vi "SQLSTATE Lookup.vi"(4 "SQLSTATE Value":string) -> (1 "SQLSTATE Description":string)   [LabVIEW 2014, in "hse-db.lvlib" / "ADO-DB-Driver.lvlib"]
uses:
  ADO-DB-Driver.lvlib
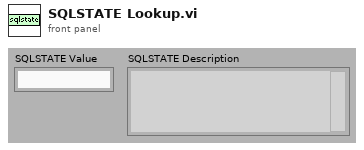
[diagram p1: front panel]
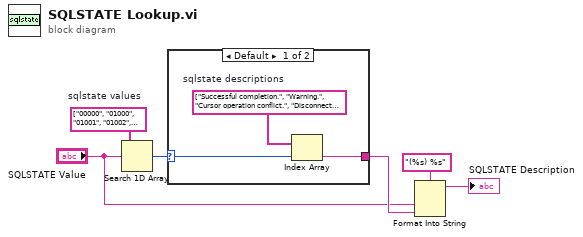
[diagram p0: block diagram]
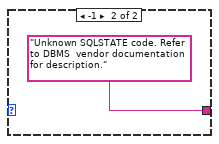
[diagram p2: hidden frame]
diagram:
  w6 = string[] ["00000", "01000", "01001", "01002", "01003", "01004", "01006", "01007", "01008", "01009", "0100A", "0100C", "0100D", "0100E", "01503", "01504", "01505", "01506", "01515", "01517", "01519", "01520", "01522", "01526", "01528", "01532", "01534", "01535", "01536", "01539", "01542", "01544", "01545", "01547", "01548", "01557", "01564", "01565", "01567", "01587", "01593", "01594", "01627", "01634", "01643", "01646", "01647", "01658", "01660", "01662", "02000", "02001", "07000", "07001", "07002", "07003", "07004", "07005", "07006", "07007", "07008", "07009", "08000", "08001", "08002", "08003", "08004", "08006", "08007", "09000", "0A000", "0A001", "0E000", "0F001", "0K000", "0W000", "0Z001", "0Z002", "20000", "21000", "22000", "22001", "22002", "22003", "22004", "22005", "22006", "22007", "22008", "22009", "22011", "22012", "22015", "22018", "22019", "22021", "22022", "22023", "22024", "22025", "22026", "22027", "22501", "22503", "22504", "22511", "22522", "22524", "22525", "23000", "23001", "23502", "23503", "23504", "23505", "23511", "23512", "23513", "23515", "23520", "23522", "24000", "24501", "24502", "24504", "24506", "24507", "24513", "24514", "25000", "25006", "25501", "26000", "26501", "26510", "27000", "28000", "2A000", "2B000", "2C000", "2D000", "2E000", "2D522", "2D528", "2D529", "2E000", "2F002", "2F003", "2F004", "2F005", "33000", "34000", "35000", "36001", "37000", "38001", "38002", "38003", "38004", "38501", "39004", "3B001", "3B002", "3B501", "3B502", "3C000", "3D000", "3F000", "40000", "40001", "40002", "40003", "42000", "42501", "42502", "42506", "42601", "42602", "42603", "42604", "42605", "42606", "42607", "42609", "42610", "42611", "42612", "42613", "42614", "42615", "42616", "42617", "42618", "42620", "42621", "42622", "42623", "42625", "42629", "42631", "42701", "42702", "42703", "42704", "42705", "42707", "42709", "42710", "42711", "42712", "42713", "42718", "42723", "42724", "42725", "42726", "42732", "42733", "42734", "42736", "42737", "42738", "42802", "42803", "42804", "42805", "42806", "42807", "42808", "42809", "42810", "42811", "42812", "42813", "42814", "42815", "42816", "42817", "42818", "42819", "42820", "42821", "42822", "42823", "42824", "42825", "42826", "42827", "42828", "42829", "42830", "42832", "42833", "42834", "42835", "42836", "42837", "42841", "42842", "42845", "42846", "42847", "42848", "42850", "42851", "42852", "42854", "42855", "42857", "42858", "42860", "42862", "42863", "42866", "42872", "42873", "42874", "42875", "42876", "42877", "42878", "42879", "42880", "42881", "42882", "42883", "42884", "42885", "42886", "42887", "42888", "42889", "42890", "42891", "42892", "42893", "42894", "42895", "42896", "42898", "42899", "428A1", "428B3", "428B7", "428B8", "428BA", "428C1", "428C7", "428C9", "428D1", "428D2", "428D4", "428D5", "428D6", "428D7", "428D8", "428EC", "428EK", "428EW", "428F1", "428F2", "428F9", "428FA", "428FC", "428FD", "428FE", "428FR", "428FT", "428FY", "428G0", "428G2", "42903", "42904", "42906", "42907", "42908", "42910", "42911", "42912", "42914", "42917", "42918", "42919", "42922", "42923", "42924", "42926", "42929", "42930", "42932", "42937", "42939", "42944", "42961", "42962", "42969", "42970", "42971", "42972", "42977", "42978", "42981", "42984", "42985", "42987", "42990", "42995", "42996", "42998", "42999", "429B6", "429B7", "429BD", "429BH", "429BM", "44000", "46001", "46002", "46003", "46007", "46008", "46501", "51002", "51003", "51004", "51009", "51015", "51021", "51035", "51036", "51037", "51039", "53038", "53039", "53045", "54001", "54002", "54004", "54005", "54006", "54008", "54009", "54010", "54011", "54018", "54019", "54021", "54023", "54028", "54035", "54038", "54044", "54054", "55005", "55006", "55007", "55018", "55019", "55029", "55042", "55048", "55050", "56016", "56084", "56095", "560BF", "560C4", "57005", "57006", "57007", "57011", "57012", "57013", "57014", "57017", "57033", "57042", "57043", "57050", "58003", "58004", "58008", "58009", "58010", "58011", "58012", "58014", "58015", "58016", "58017", "58018", "58028", "58033", "60000", "61000", "62000", "63000", "64000", "65000", "66000", "67000", "69000", "72000", "82100", "82101", "82102", "82103", "82104", "82105", "82106", "82107", "82108", "82109", "82110", "82111", "82112", "82113", "82114", "82115", "82116", "82117", "82118", "82119", "82120", "82121", "82122", "90000", "99999", "HZ000"]  # sqlstate values
  n1 = Search 1D Array(1D array=w6, element="SQLSTATE Value") -> (index of element=w1:i32)  [unwired: 1 in]
  n2 = case shown="Default" w1 {
    selector: w1 -> [w7 _]
    tunnel: [w8 "Unknown SQLSTATE code. Refer to DBMS  vendor documentation for description."] -> w5
    frame Default {
      w9 = string[] ["Successful completion.", "Warning.", "Cursor operation conflict.", "Disconnect error.", "Null value eliminated in set function.", "The value of a string was truncated when assigned to another string data type with a shorter length.", "Privilege not revoked.", "Privilege not granted.", "Implicit zero-bit padding.", "Search condition too long for information schema.", "Query expression too long for information schema.", "One or more ad hoc result sets were returned from the procedure.", "The cursor that was closed has been reopened on the next result set within the chain.", "The procedure returned too many result sets.", "The number of result columns is larger than the number of host variables provided.", "The update or delete statement does not include a where clause.", "The statement was not executed because it is unacceptable in this environment.", "An adjustment was made to a date or timestamp value to correct an invalid date resulting from an arithmetic operation.", "The null value has been assigned to a host variable, because the non-null value of the column is not within the range of the host variable.", "A character that cannot be converted was replaced with a substitute character.", "The null value has been assigned to a host variable, because a numeric value is out of range.", "The null value has been assigned to a host variable, because the characters cannot be converted.", "The local table or view name used in the \"create alias\" statement is undefined.", "Isolation level has been escalated.", "Where not null is ignored, because the index key cannot contain null values.", "An undefined object name was detected.", "The string representation of a datetime value is invalid.", "An arithmetic operation on a date or timestamp has a result that is not within the valid range of dates.", "During remote bind where existence checking is deferred, the server-name specified does not match the current server.", "Connection is successful but only sbcs characters should be used.", "Authorization id does not have the privilege to perform the operation as specified.", "The null value has been assigned to a host variable, because a substring error occurred; for example, an argument of substr is out of range.", "An unqualified column name has been interpreted as a correlated reference.", "A mixed data value is improperly formed.", "The authorization id does not have the privilege to perform the specified operation on the identified object.", "Too many host variables have been specified on select into or fetch.", "The null value has been assigned to a host variable, because division by zero occurred.", "The null value has been assigned to a host variable, because a miscellaneous data exception occurred; for example, the character value for the cast, decimal, float, or integer scalar function is invalid; a floating-point NaN (not a number) or invalid data in a packed decimal field was detected.", "The table was created but not journaled.", "The unit of work was committed or rolled back, but the outcome is not fully known at all sites.", "An alter table may cause data truncation.", "Insufficient number of entries in an SQLDA for all information (i.e. Not enough descriptors to return the distinct name).", "The datalink value may not be valid because the table is in reconcile pending or reconcile is not a possible state.", "The distinct data type name is too long and cannot be returned in the SQLDA. The short name is returned instead.", "Assignment to SQLCODE or SQLSTATE variable does not signal a warning or error.", "A result sets cannot be returned because the cursor was closed.", "A db2sql before trigger changed to db2row.", "Binary data is invalid for decrypt_char and decyrypt_db.", "The routine was created but a restore will not update the catalog.", "Release record option ignored on close.", "No data found.", "No additional result sets returned.", "Dynamic SQL error.", "The number of host variables is not correct for the number of parameter markers.", "The call parameter list is invalid.", "Cursor specification cannot be executed.", "Using clause required for dynamic parameters.", "Prepared statement not a cursor specification.", "Restricted datatype attribute violation.", "Using clause required for result fields.", "Invalid descriptor count.", "Invalid descriptor index.", "Connection exception.", "Client is unable to establish a connection.", "Connection name in use.", "Connection does not exist.", "The server rejected the connection.", "Connection failure.", "Transaction resolution unknown.", "A triggered SQL statement failed.", "Feature not supported.", "Multiple server transactions.", "The schema name list in a set(tm) path statement is not valid.", "The locator value does not currently represent any value.", "A resignal was issued but a handler is not active.", "The statement is not allowed in a trigger.", "Maximum number of stacked diagnostics areas exceeded.", "Stacked diagnostics accessed without and active handler.", "The case was not found for the case statement.", "The result of a select into, scalar fullselect, or subquery of a basic predicate is more than one value.", "Data exception.", "String data truncated (on right) on insert or update.", "Null value returned with no indicator variable provided.", "Numeric value out-of-range or overflow.", "A null value cannot returned from a procedure that is defined as parameter style general or a type-preserving method that is invoked with a non-null argument.", "Error in assignment.", "The fetch orientation is invalid.", "Invalid date-time format.", "Date-time field overflow.", "Invalid time zone displacement value.", "Substring error.", "Divide by zero error.", "Interval field overflow.", "Invalid character value for cast.", "Invalid escape character (in the \"like\" predicate?).", "A character is not in the coded character set or the conversion is not supported.", "Indicator variable overflow.", "Invalid parameter value.", "Unterminated C string passed as input host variable.", "Invalid escape sequence, for example, escape char not followed by %, _, or escape char.", "String data - length mismatch.", "Trim error.", "The length control field of a variable length string is negative or greater than the maximum.", "The string representation of a name is invalid.", "A mixed data value is invalid.", "ADT length exceeds maximum column length. The value for a rowid or reference column is not valid.", "A ccsid value is not valid at all, not valid for the data type or subtype, or not valid for the encoding scheme.", "Character conversion resulted in truncation.", "Partitioning key value is not valid.", "Integrity constraint violation.", "The update or delete of a parent key is prevented by a restrict update or delete rule.", "An insert or update value is null, but the column cannot contain null values.", "The insert or update value of a foreign key is invalid.", "The update or delete of a parent key is prevented by a no action update or delete rule.", "A violation of the constraint imposed by a unique index or a unique constraint occurred.", "A parent row cannot be deleted, because the check constraint restricts the deletion.", "The check constraint cannot be added, because the table contains rows that do not satisfy the constraint definition.", "The resulting row of the insert or update does not conform to the check constraint definition.", "The unique index cannot be created or unique constraint added because the table contains duplicate values of the specified key.", "The foreign key cannot be defined, because all of its values are not equal to a parent key of the parent table.", "The range of values for the identity column or sequence is exhausted.", "Invalid cursor state.", "The identified cursor is not open.", "The cursor identified in an open statement is already open.", "The cursor identified in the update, delete, set, or get statement is not positioned on a row.", "The statement identified in the prepare is the statement of an open cursor.", "Fetch current was specified, but the current row is deleted, or a value of an order by column of the current row has changed.", "Fetch next, prior, current, or relative is not allowed, because the cursor position is not known.", "A previous error has disabled this cursor.", "Invalid transaction state.", "An update operation is not valid because the transaction is read only.", "The statement is only allowed as the first statement in a unit of work.", "Invalid SQL statement name.", "The statement identified does not exist.", "The statement name specified in a declare cursor already has a cursor allocated to it.", "Triggered data change violation.", "Invalid authorization specification.", "Direct SQL syntax error or access rule violation.", "Dependent privilege descriptors still exist.", "Invalid character set name.", "Invalid transaction termination.", "Invalid connection name.", "Commit and rollback are not allowed in an atomic compound statement.", "Dynamic commit or commit on return procedure is invalid for the application execution environment.", "Dynamic rollback is invalid for the application execution environment.", "Connection name is invalid.", "The SQL function attempted to modify data, but the function was not defined as modifies SQL data.", "The statement is not allowed in a function or procedure.", "The SQL function attempted to read data, but the function was not defined as reads SQL data.", "The function did not execute a return statement.", "Invalid SQL descriptor name.", "Invalid cursor name.", "Invalid condition number.", "A sensitive cursor cannot be defined for the specified select-statement.", "Dynamic SQL syntax error or access rule violation.", "The external routine is not allowed to execute SQL statements.", "The external routine attempted to modify data, but the routine was not defined as modifies SQL data.", "The statement is not allowed in a routine.", "The external routine attempted to read data, but the routine was not defined as reads SQL data.", "Error occurred while calling a user-defined function, external procedure, or trigger (using the simple call or simple call with nulls calling convention).", "A null value is not allowed for an in or inout argument when using parameter style general or an argument that is a java(tm) primitive type.", "The savepoint is not valid.", "The maximum number of savepoints has been reached.", "A duplicate savepoint name was detected.", "A release or rollback to savepoint was specified, but a savepoint does not exist.", "Ambiguous cursor name.", "Invalid catalog name.", "Invalid schema name.", "Transaction rollback.", "Serialization failure. Transaction rollback due to deadlock.", "Integrity constraint violation.", "Statement completion unknown.", "Syntax error or access rule violation.", "The authorization id does not have the privilege to perform the specified operation on the identified object.", "The authorization id does not have the privilege to perform the operation as specified.", "Owner authorization failure occurred.", "A character, token, or clause is invalid or missing.", "A character that is invalid in a name has been detected.", "An unterminated string constant has been detected.", "An invalid numeric or string constant has been detected.", "The number of arguments specified for a scalar function is invalid.", "An invalid hexadecimal constant has been detected.", "An operand of a column function or concat operator is invalid.", "All operands of an operator or predicate are parameter markers.", "A parameter marker is not allowed.", "The column or argument definition is invalid.", "The statement string is an SQL statement that is not acceptable in the context in which it is presented.", "Clauses are mutually exclusive.", "A duplicate keyword or clause is invalid.", "An invalid alternative was detected.", "Invalid options are specified.", "The statement string is blank or empty.", "A host variable is not allowed.", "Read-only scroll was specified with the update clause.", "The check constraint generated column expression is invalid.", "A name or label is too long.", "A default clause cannot be specified.", "A case expression is invalid.", "Parameter names must be specified for SQL routines.", "An expression must be specified on a return statement in an SQL function.", "A duplicate column name in an insert or update operation or the set transition-variable was detected.", "A column reference is ambiguous, because of duplicate names.", "An undefined column or parameter name was detected.", "An undefined object or constraint name was detected.", "An undefined server-name was detected.", "A column name in order by does not identify a column of the result table.", "A duplicate column name was specified in a key column list.", "A duplicate object or constraint name was detected.", "A duplicate column name was detected in the object definition or alter table statement.", "A duplicate table designator was detected in the from clause or referencing clause of a create trigger statement.", "A duplicate object was detected in a list or is the same as an existing object.", "The local server name is not defined.", "A function with the same signature already exists in the schema.", "Unable to access an external program used for a user-defined function or a procedure.", "A routine or method was referenced directly (not by either signature or by specific instance name), but there is more than one specific instance of that routine or method.", "Duplicate names for common table expressions were detected.", "A duplicate schema name in the set current path statement was detected.", "A procedure with the specified name cannot be added to the schema because the procedure overloading is not allowed in this database and there is already a procedure with the same name in the schema.", "A duplicate parameter-name, SQL variable name, label, or condition-name was detected.", "The label specified on the goto, iterate, or leave statement is not found or not valid.", "The condition specified is not defined.", "A duplicate column name or unnamed column was specified in a declare cursor statement of a for statement.", "The number of insert or update values is not the same as the number of columns.", "A column reference in the select or having clause is invalid, because it is not a grouping column; or a column reference in the group by clause is invalid.", "The result expressions in a case expression are not compatible.", "An integer in the order by clause does not identify a column of the result table.", "A value cannot be assigned to a host variable, because the data types are not compatible.", "The insert, update, or delete is not permitted on this object.", "A column identified in the insert or update operation is not updateable.", "The identified object is not the type of object to which the statement applies.", "A base table is not identified in a foreign key clause.", "The number of columns specified is not the same as the number of columns in the select clause.", "A library name is required in create table in the system-naming mode.", "With check option cannot be used for the specified view.", "The column cannot be dropped, because it is the only column in the table.", "The data type, length, scale, value, or ccsid is invalid.", "A datetime value or duration in an expression is invalid.", "The column cannot be dropped, because restrict was specified and a view or constraint is dependent on the column or the column is part of a partitioning key.", "The operands of an operator or function are not compatible.", "An operand of an arithmetic operation or an operand of a function that requires a number is not a number.", "A numeric constant is too long, or it has a value that is not within the range of its data type.", "A data type for an assignment to a column or variable is not compatible with the data type.", "An expression in the order by clause or group by clause is not valid.", "Multiple columns are returned from a subquery that only allows one column.", "An operand of like is not a string, or the first operand is not a column.", "The rows of union, intersect, except, or values do not have compatible columns.", "The rows of union, intersect, except, or values do not have the same number of columns.", "The table identified in the update or delete is not the same table designated by the cursor.", "The table designated by the cursor of the update or delete statement cannot be modified, or the cursor is read-only.", "For update of is invalid, because the result table designated by the cursor cannot be modified.", "The foreign key does not conform to the description of the parent key.", "The operation is not allowed on system objects.", "The qualified object name is inconsistent with the naming option.", "Set null cannot be specified, because no column of the foreign key can be assigned the null value.", "Cyclic references cannot be specified between named derived tables.", "The specification of a recursive, named derived table is invalid.", "The column cannot be altered, because its attributes are not compatible with the current column attributes.", "A parameter marker can not be a user-defined type or reference type.", "A column or parameter definition is invalid, because a specified option is inconsistent with the column description.", "An invalid use of a not deterministic or external action function was detected.", "Cast from source type to target type is not supported.", "An ovrdbf command was issued for one of the referenced files, but one of the parameters is not valid for SQL.", "Isolation level cs with keep locks is not allowed.", "A logical file is invalid in create view.", "A referenced file is not a table, view, or physical file.", "The privileges specified in grant or revoke are invalid or inconsistent. (for example, grant alter on a view.).", "A result column data type in the select list is not compatible with the defined type in a typed view or materialized query table definition.", "The assignment of the lob to this host variable is not allowed. The target host variable for all fetches of this lob value for this cursor must be a locator or lob variable.", "A referenced file has more than one format.", "Operation cannot be applied to the specified object.", "The constraint cannot be dropped because it is enforcing a primary key or rowid.", "An extended dynamic statement cannot be executed against a non-extended dynamic package.", "An undefined host variable in rexx has been detected.", "The data type in either the returns clause or the cast from clause in the create function statement is not appropriate for the data type returned from the source function or return statement in the function body.", "Fetch statement clauses are incompatible with the cursor definition.", "An invalid number of rows was specified in a multiple-row fetch or multiple-row insert.", "ALWCPYDTA(*no) was specified, but a copy is necessary to implement the select-statement.", "The schema-name portion of a qualified name must be the same name as the schema name.", "Different ccsids for keys in create index are only allowed with a *hex sort sequence.", "The column name cannot be qualified.", "An invalid function or procedure name was used with the external keyword.", "The data type of one or more input parameters in the create function statement is not appropriate for the corresponding data type in the source function.", "The cast to and cast from data types are incompatible, or would always result in truncation of a fixed string.", "Invalid use of a function.", "The specific instance name qualifier is not equal to the function name qualifier.", "No function or method was found with a matching signature.", "No routine was found with the specified name and compatible arguments.", "The number of input parameters specified on a create function statement does not match the number provided by the function named in the source clause.", "The in, out, or inout parameter attributes do not match.", "The function is not valid in the context where it occurs.", "The table does not have a primary key.", "The table already has a primary key.", "A column list was specified in the references clause, but the identified parent table does not have a unique constraint with the specified column names.", "A duplicate unique constraint already exists.", "The referential constraint and trigger are not allowed, because the delete rule and trigger event are not compatible.", "The object or constraint cannot be dropped or authorities cannot be revoked from the object, because other objects are dependent on it.", "The value of a column or sequence attribute is invalid.", "For static SQL, an input host variable cannot be used, because its data type is not compatible with the parameter of a procedure or user-defined function.", "The asp number is invalid.", "An invalid correlated reference or transition table was detected in a trigger.", "Correlated references and column names are not allowed for triggered actions with the for each statement clause.", "Unable to access a file referenced by a file reference variable.", "An invalid SQLSTATE was specified.", "A number specified in an SQL statement is out of the valid range.", "The name specified on a rename is not valid.", "Without return cursors must not be specified in set result sets.", "Only one rowid or identity column can be specified for a table.", "A rowid or reference column specification is not valid.", "A rowid or identity column cannot be specified as the target column of an insert or update.", "Unable to access a file referenced by a datalink value.", "As locator cannot be specified for a non-lob parameter.", "A cursor specified in a for statement cannot be referenced in an open, close, or fetch statement.", "The ending label does not match the beginning label.", "Undo is not allowed for not atomic compound statements.", "The condition value is not allowed.", "The SQLCODE or SQLSTATE variable declaration is not valid.", "The fullselect specified for the materialized query table is not valid.", "The qualifier for a declared global temporary table name or an index on a declared global temporary table must be session.", "The table cannot be converted to or from a materialized query table.", "An SQL table function must return a table result.", "An integer expression must be specified on a return statement in an SQL procedure.", "A sequence expression cannot be specified in this context.", "The scale of the decimal number must be zero.", "The length of the encryption password is not valid.", "The password used for decryption does not match the password used to encrypt the data.", "The data is not a result of the encrypt function.", "A column cannot be altered as specified.", "The table is not compatible with the specified data partitioning operation.", "A column cannot be added, dropped, or altered in a materialized query table.", "A logical file prevents the alter of the partition attributes.", "The last data partition cannot be dropped from the table.", "Invalid use of an aggregate function or OLAP function.", "The SQL procedure was not created because of a compile error.", "A column function in a subquery of a having clause includes an expression that applies an operator to a correlated reference.", "The string is too long.", "The statement does not include a required column list.", "The statement is not allowed in a compound statement.", "A decimal divide operation is invalid, because the result would have a negative scale.", "A column cannot be updated, because it is not identified in the update clause of the select-statement of the cursor.", "The delete is invalid, because a table referenced in a subquery can be affected by the operation.", "The object cannot be explicitly dropped or altered.", "A user-defined data type cannot be created with a system-defined data type name (for example, integer).", "Nested compound statements are not allowed.", "Drop schema cannot be executed under commitment control.", "Program or package must be recreated to reference an alias-name.", "An alias resolved to another alias rather than a table or view at the remote location.", "Locators are not allowed with commit(*none).", "For all partitions is not allowed for an encoded vector index.", "The same column was identified in for update of and order by.", "The program preparation assumptions are incorrect.", "The parameter must not have a subtype of mixed.", "The name cannot be used, because the specified identifier is reserved for system use.", "The authorization id cannot be both an owner and primary group owner.", "The server name specified does not match the current server.", "A long column, lob column, structured type column or datalink column cannot be used in an index, a key, or a constraint.", "The package was not created and the current unit of work was rolled back, because of internal limitations or an invalid section number.", "Commit hold or rollback hold is only allowed to a db2 udb for iseries application server.", "SQL statements cannot be executed under commitment control, because commitment control is already active to another relational database.", "An expression in a join-condition or on clause of a merge statement references columns in more than one of the operand tables.", "The authorization id cannot be changed when connecting to the local server.", "An indicator variable is not a small integer.", "Create schema is not allowed if changes are pending in the unit of work.", "The privilege cannot be granted to the view, because *objopr or *objmgt authority exists on a dependent view or table, and the grantee does not have *allobj or the specified privilege on the dependent table or view.", "The statement is not allowed in a routine.", "The statement is not allowed in a trigger.", "A unique index or unique constraint is not allowed because the key columns are not a superset of the partitioned key columns.", "The requested function does not apply to global temporary tables.", "The partition key cannot be a datetime or floating-point column.", "A referential constraint is not allowed because the foreign key columns are not a superset of the partitioned key columns or the node group is not the same as the parent table.", "The query is not allowed on a distributed table or view.", "Rows from a distributed table cannot be redistributed because the table contains a datalink column with file link control.", "A referential constraint with a delete rule of cascade is not allowed on a table with a datalink column with file link control.", "Return must be the last SQL statement of the atomic compound statement within an SQL row or table function.", "A partitioned table cannot contain an identity column.", "The icu sort sequence cannot be used in this context.", "View with check option violation.", "The url specified on an install or replace of a jar procedure did not identify a valid jar file.", "The jar name specified on the install, replace, or remove of a java procedure is not valid.", "The jar file cannot be removed, a class is in use by a procedure.", "A java function has a java method with an invalid signature.", "A java function cannot map to a single java method.", "The install or remove jar procedure for \"<jar-id>\" specified the use of a deployment descriptor.", "The package corresponding to an SQL statement execution request was not found.", "Consistency tokens do not match.", "An address in the SQLDA is invalid.", "Commit or rollback is not allowed, because commitment control has not been started.", "An attempt was made to execute a section that was found to be in error at bind time.", "SQL statements cannot be executed until the application process executes a rollback operation.", "A prevval expression cannot be used because a value has not been generated for the sequence yet in this session.", "An implicit connect to a remote server is not allowed because a savepoint is outstanding.", "The operation is not allowed because a trigger has been marked inoperative.", "The encryption password value is not set.", "The number of key limit values is zero or greater than the number of columns in the key.", "The part clause of the alter statement is omitted or invalid.", "The data type of the key limit constant is not the same as the data type of the column.", "The statement is too long or too complex.", "A string constant is too long.", "The statement has too many table names or too many items in a select or insert list.", "The sort key is too long, or has too many columns.", "The result of concatenation is too long.", "The key is too long, a column of the key is too long, or the key many columns.", "Too many users were specified in grant or revoke.", "The record length of the table is too long.", "Too many columns were specified for a table, view, or table function.", "The row is too long.", "The maximum number of late descriptors has been exceeded, probably because too many different ccsids were used.", "Too many constraints, or the size of the constraint is too large.", "The limit for the number of parameters or arguments for a function or a procedure has been exceeded.", "The maximum number of concurrent lob handles has been reached.", "An internal object limit exceeded.", "Maximum depth of nested routines or triggers was exceeded.", "A multiple-byte (ucs-2) sort sequence table cannot be supported in drda(r) because it is too large.", "The combination of the number of table space partitions and the corresponding length of the partitioning limit key it too large.", "Recursion is only supported to a db2 udb for iseries application server.", "The object cannot be dropped, because it is currently in use by the same application process.", "The object cannot be altered, because it is currently in use by the same application process.", "The schema cannot be dropped, because it is in the library list.", "The object is in an invalid state for the operation.", "Local program attempted to connect to a remote database.", "The alias is not allowed because it identifies a single member of a multiple member file.", "Encrypted data cannot be encrypted.", "An object cannot be created into a protected schema.", "The ranges specified for data partitions are not valid.", "An unsupported sqltype was encountered in a select list or input list.", "A bind option is invalid.", "The encryption and decryption facility has not been installed.", "The option is not valid for the ard interface.", "The statement cannot be executed, because a utility or a governor time limit was exceeded.", "The object cannot be created, because a drop or create is pending.", "The object cannot be used, because an operation is pending.", "Virtual storage or database resource is not available.", "A non-database resource is not available. This will not affect the successful execution of subsequent statements.", "A non-database resource is not available. This will affect the successful execution of subsequent statements.", "Processing was canceled as requested.", "Character conversion is not defined.", "Deadlock or timeout occurred without automatic rollback.", "DDM recursion has occurred.", "A local SQL application program cannot be executed on an application server.", "The file server is not currently available.", "An invalid section number was detected.", "A system error (that does not necessarily preclude the successful execution of subsequent SQL statements) occurred.", "Execution failed due to a distribution protocol error that will not affect the successful execution of subsequent DDM commands or SQL statements.", "Execution failed due to a distribution protocol error that caused deallocation of the conversation.", "Execution failed due to a distribution protocol error that will affect the successful execution of subsequent DDM commands or SQL statements.", "The DDM command is invalid while the bind process in progress.", "The bind process with the specified package name and consistency token is not active.", "The DDM command is not supported.", "The DDM object is not supported.", "The DDM parameter is not supported.", "The DDM parameter value is not supported.", "The DDM reply message is not supported.", "The commit operation failed, because a resource in the unit of work was not able to commit its resources.", "An unexpected error occurred while attempting to access a client driver.", "System errors.", "Resource error.", "Multi-threaded server and detached process errors.", "Oracle*xa and two-task interface errors.", "Control file, database file, and redo file errors; archival and media recovery errors.", "PL/SQL errors.", "SQL*net driver errors.", "Licensing errors.", "SQL*connect errors.", "SQL execute phase errors.", "Out of memory (could not allocate).", "Inconsistent cursor cache: unit cursor/global cursor mismatch.", "Inconsistent cursor cache: no global cursor entry.", "Inconsistent cursor cache: out of range cursor cache reference.", "Inconsistent host cache: no cursor cache available.", "Inconsistent cursor cache: global cursor not found.", "Inconsistent cursor cache: invalid oracle cursor number.", "Program too old for runtime library.", "Invalid descriptor passed to runtime library.", "Inconsistent host cache: host reference is out of range.", "Inconsistent host cache: invalid host cache entry type.", "Heap consistency error.", "Unable to open message file.", "Code generation internal consistency failed.", "Reentrant code generator gave invalid context.", "Invalid hstdef argument.", "First and second arguments to sqlrcn both null.", "Invalid open or prepare for this connection.", "Application context not found.", "Connect error; can't get error text.", "Precompiler/sqllib version mismatch.", "Fetched number of bytes is odd.", "Exec tools interface is not available.", "Debug events.", "Catch all.", "Remote database access."]  # sqlstate descriptions
      n3 = Index Array(array=w9, index=w7) -> (element=w8:string)
    }
    frame -1 {
    }
  }
  n4 = Format Into String(format string="(%s) %s", "SQLSTATE Value", w5) -> (resulting string=→"SQLSTATE Description":string)  [unwired: 2 in, 1 out]
